vi "Rohde & Schwarz VNA Initialize.vi"(8 "error in (no error)":errorcluster, 11 "Configuration":T2={"BusType"=enum."GPIB", "GPIB Bus"=0, "GPIB Address"=16, "IP"=0, "COM"=1, "Baud Rate"=enum."9600", "USB Device"=0, "Instrument S\\N"="", "SCIL Address"=16} {"USB Device" max=31 step=1}) -> (0 "error out":errorcluster {"code" format="%.0x"}, 3 "dup VISA Resource Name":refnum<visa-resource-name>, 5 "Rohde & Schwarz VNA":T1)   [LabVIEW 2011]
uses:
  VNA Configuration.ctl
  TypeDefs/Rohde & Schwarz VNA Instrument Info.ctl
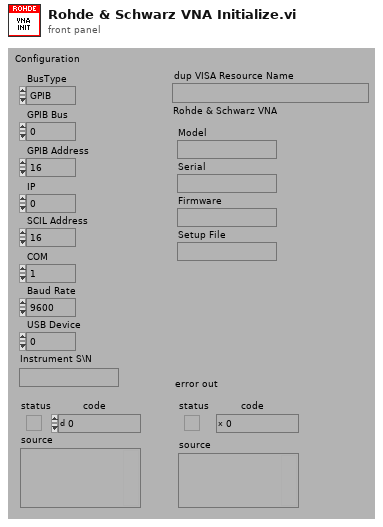
[diagram p1: front panel]
types:
  T1 = typedef "Rohde & Schwarz VNA Instrument Info.ctl" = cluster{"Model":string, "Serial":string, "Firmware":string, "Setup File":string}
  T2 = typedef "VNA Configuration.ctl" = cluster{"BusType":enum32{"GPIB", "LAN/IP", "Serial", "USB"}, "GPIB Bus":i32, "GPIB Address":i32, "IP":u32, "COM":i32, "Baud Rate":enum32{"300", "600", "1200", "2400", "4800", "9600"}, "USB Device":u32, "Instrument S\\N":string, "SCIL Address":i32}
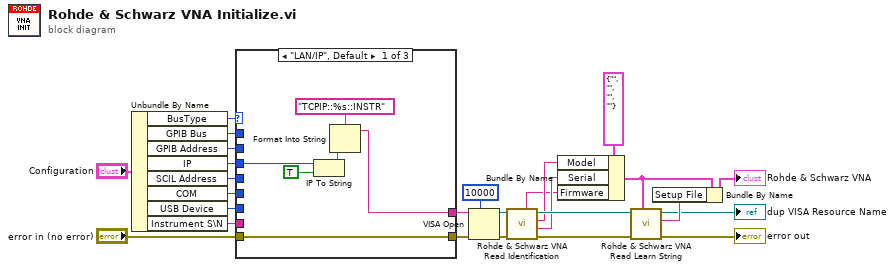
[diagram p0: block diagram]
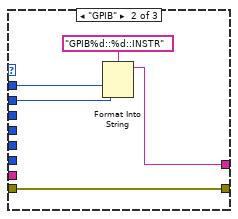
[diagram p2: hidden frame]
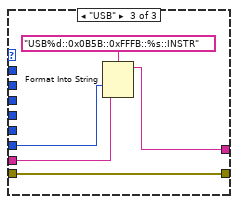
[diagram p3: hidden frame]
diagram:
  n1 = Unbundle By Name("Configuration") -> ("BusType"=w25:enum32{"GPIB", "LAN/IP", "Serial", "USB"}, "GPIB Bus"=w24:i32, "GPIB Address"=w23:i32, "IP"=w21:u32, "SCIL Address"=w2:i32, "COM"=w1:i32, "USB Device"=w20:u32, "Instrument S\\N"=w4:string)
  n2 = case shown="\"LAN/IP\", Default" w25 {
    tunnel: "error in (no error)" -> [w28 w37 w40]
    tunnel: w24 -> [_ w35 _]
    tunnel: w23 -> [_ w34 _]
    tunnel: [w27 w33 w39] -> w3
    tunnel: [w28 w37 w40] -> w8
    tunnel: w21 -> [w29 _ _]
    tunnel: w20 -> [_ _ w41]
    tunnel: w4 -> [_ _ w38]
    tunnel: w2 -> [_ _ _]
    tunnel: w1 -> [_ _ _]
    frame "LAN/IP", Default {
      n3 = IP To String(1:TRUE ("dot notation? (F)"), 2:w29) -> (0:w31:string)
      n4 = Format Into String(format string="TCPIP::%s::INSTR", w31) -> (resulting string=w27:string)  [unwired: 2 in, 1 out]
    }
    frame "GPIB" {
      n5 = Format Into String(format string="GPIB%d::%d::INSTR", w35, w34) -> (resulting string=w33:string)  [unwired: 2 in, 1 out]
    }
    frame "USB" {
      n6 = Format Into String(format string="USB%d::0x0B5B::0xFFFB::%s::INSTR", w41, w38) -> (resulting string=w39:string)  [unwired: 2 in, 1 out]
    }
  }
  n7 = VISA Open(timeout (0)=u32 10000 ("VISA Open timeout (0)"), error in (no error)=w8, VISA resource name=w3) -> (VISA resource name=w18:refnum<visa-resource-name>, error out=w19:errorcluster)  [unwired: 2 out]
  n8 = call "Rohde & Schwarz VNA Read Identification.vi"("error in (no error)"=w19, "VISA Resource Name"=w18) -> ("error out"=w15:errorcluster, "Serial Number"=w13:string, "Model Number"=w12:string, "dup VISA Resource Name"=w14:refnum<visa-resource-name>, "Firmware"=w11:string)  [unwired: 5 out]
  n9 = Bundle By Name(cluster=T1 {"Model"="", "Serial"="", "Firmware"="", "Setup File"=""} ("Rohde & Schwarz VNA"), "Model"=w12, "Serial"=w13, "Firmware"=w11) -> (w16:T1)
  n10 = call "Rohde & Schwarz VNA Read Learn String.vi"("Rohde & Schwarz VNA"=w16, "error in (no error)"=w15, "VISA Resource Name"=w14) -> ("error out"=→"error out":errorcluster, "Learn String"=w17:string, "dup VISA Resource Name"=→"dup VISA Resource Name":refnum<visa-resource-name>)  [unwired: 6 out]
  n11 = Bundle By Name(cluster=w16, "Setup File"=w17) -> (→"Rohde & Schwarz VNA":T1)
